vi "SwitchOption.vi"(6 "SubPanelRef":refnum<vi>, 7 "Panel Controller":refnum<class "MemberPanel.lvclass">, 8 "error in (no error)":errorcluster, 9 "Base Path":path, 10 "ThreadName(\"\")":string, 11 "Member_Actor in":refnum<class "Member_Actor.lvclass">) -> (0 "error out":errorcluster, 3 "Member_Actor out":refnum<class "Member_Actor.lvclass">)   [LabVIEW 2015, in "Member_Actor.lvlib" / "Member_Actor.lvclass"]
uses:
  Member_Actor.lvclass
  MemberPanel/MemberPanel.lvclass
  Member_Actor.lvclass/Member_Actor.ctl
  SubPanel/ExcuseNote_Panel.vi
  SubPanel/Information_Panel.vi
  SubPanel/TimeTable_Panel.vi
  Member_Actor.lvlib
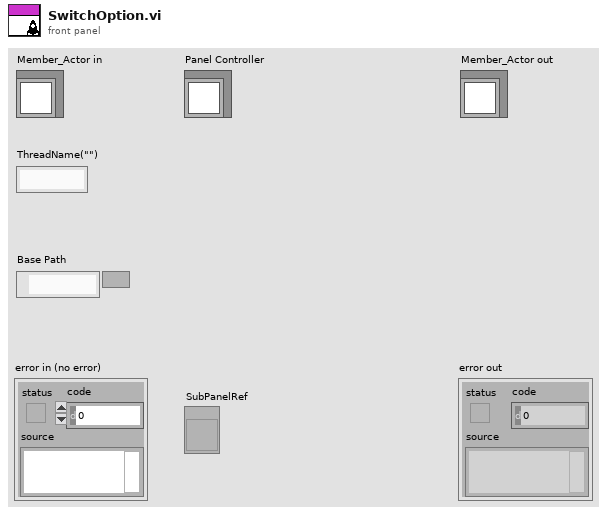
[diagram p1: front panel]
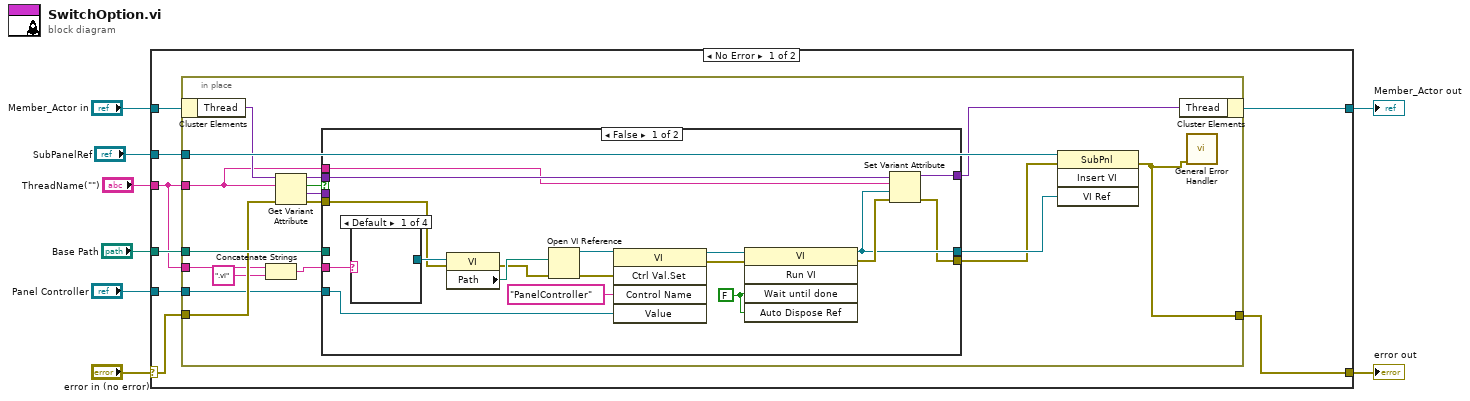
[diagram p0: block diagram]
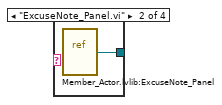
[diagram p2: hidden frame]
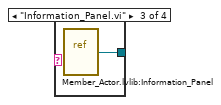
[diagram p3: hidden frame]
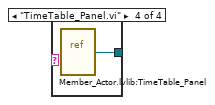
[diagram p4: hidden frame]
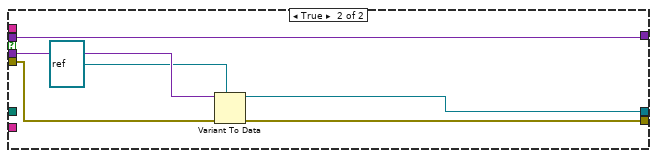
[diagram p5: hidden frame]
diagram:
  n1 = case shown="No Error" "error in (no error)" {
    selector: "error in (no error)" -> [w11 w62]
    tunnel: [w14 w62] -> w7
    tunnel: [w10 w61] -> w5
    tunnel: "Member_Actor in" -> [w13 w61]
    tunnel: "Base Path" -> [w16 _]
    tunnel: "ThreadName(\"\")" -> [w12 _]
    tunnel: "SubPanelRef" -> [w15 _]
    tunnel: "Panel Controller" -> [w9 _]
    frame No Error {
      n2 = in-place {
        in-place-border: w16 -> [w33]
        in-place-border: w12 -> [w21]
        in-place-border: w15 -> [w32]
        in-place-border: [w18] -> w14
        in-place-border: w12 -> [w17]
        in-place-border: w11 -> [w28]
        in-place-border: w9 -> [w22]
        n3 = in-place-cluster #1(w13) -> ("Thread"=w29:variant)
        n4 = Concatenate Strings(w21, ".vi" ("string")) -> (w19:string)
        n5 = Get Variant Attribute(Variant=w29, name=w17, error in=w28) -> (duplicate Variant=w25:variant, found=w27:bool, value=w24:variant, error out=w26:errorcluster)  [unwired: 1 in]
        n6 = case shown="False" w27 {
          tunnel: w33 -> [_ _]
          tunnel: w19 -> [w38 _]
          tunnel: [w48 w57] -> w31
          tunnel: [w47 w56] -> w30
          tunnel: w26 -> [w36 w59]
          tunnel: w25 -> [w50 w55]
          tunnel: [w46 w55] -> w23
          tunnel: w24 -> [_ w60]
          tunnel: w22 -> [w40 _]
          tunnel: w17 -> [w39 _]
          frame False {
            w51 = FALSE ("Wait Until Done")
            n7 = case shown="Default" w38 {
              tunnel: [_ w52 w53 w54] -> w37
              frame Default {
              }
              frame "ExcuseNote_Panel.vi" {
                n8 = vi-ref "Member_Actor.lvlib:ExcuseNote_Panel.vi"() -> (w52:refnum<vi>)
              }
              frame "Information_Panel.vi" {
                n9 = vi-ref "Member_Actor.lvlib:Information_Panel.vi"() -> (w53:refnum<vi>)
              }
              frame "TimeTable_Panel.vi" {
                n10 = vi-ref "Member_Actor.lvlib:TimeTable_Panel.vi"() -> (w54:refnum<vi>)
              }
            }
            n11 = property class="VI"(reference=w37, error in=w36) -> (error out=w34:errorcluster, "Path"=w35:path)  [unwired: 1 out]
            n12 = Open VI Reference(vi path=w35, error in (no error)=w34) -> (vi reference=w45:refnum<vi>, error out=w44:errorcluster)  [unwired: 4 in]
            n13 = invoke class="VI" method="Ctrl Val.Set"(reference=w45, error in=w44, "Control Name"="PanelController", "Value"=w40) -> (reference out=w42:refnum<vi>, error out=w43:errorcluster)  [unwired: 1 in, 3 out]
            n14 = invoke class="VI" method="Run VI"(reference=w42, error in=w43, "Wait until done"=w51, "Auto Dispose Ref"=w51) -> (reference out=w48:refnum<vi>, error out=w49:errorcluster)  [unwired: 1 in, 3 out]
            n15 = Set Variant Attribute(Variant=w50, name=w39, value=w48, error in=w49) -> (Variant out=w46:variant, error out=w47:errorcluster)  [unwired: 1 out]
          }
          frame True {
            n16 = Variant To Data(error in=w59, type=refnum<vi> refnum ("vi reference"), Variant=w60) -> (data=w57:refnum<vi>, error out=w56:errorcluster)
          }
        }
        n17 = invoke class="SubPnl" method="Insert VI"(reference=w32, error in=w30, "VI Ref"=w31) -> (error out=w18:errorcluster)  [unwired: 1 in, 3 out]
        n18 = in-place-cluster #1("Thread"=w23) -> (w10:refnum<class "Member_Actor.lvclass">)
        n19 = call <vilib>:"General Error Handler.vi"("error in (no error)"=w18) -> ()  [unwired: 10 in, 5 out]
      }
    }
    frame Error {
    }
  }
  "error out" <- w7
  "Member_Actor out" <- w5
